vi "Start and End to Array 2.vi"(6 "Sweep Style":enum16{"Linear Step", "Linear Pts", "Log Pts"}(ring), 8 "Round Factor":dbl=1000000000.0, 9 "Step or # Pts":dbl=0.1, 10 "End":dbl=2.0, 11 "Start":dbl=-0.5) -> (3 "Array":dbl[](array[numeric])=[-0.5, -0.4, -0.3, -0.2, -0.1, 0.0, 0.1, 0.2, 0.3, 0.4, 0.5, 0.6, 0.7, 0.8, 0.9, 1.0, 1.1, 1.2, 1.3, 1.4, 1.5, 1.6, 1.7, 1.8, 1.9, 2.0])   [LabVIEW 2010]
panel:
  in  "Array Settings":T1
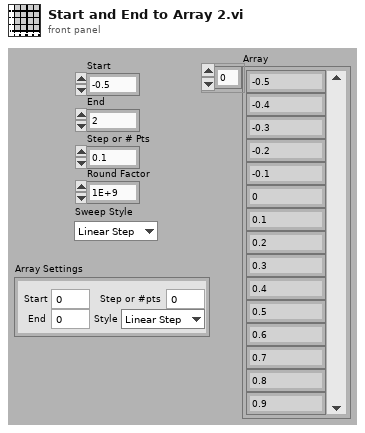
[diagram p1: front panel]
types:
  T1 = cluster{"Start":dbl, "End":dbl, "Step or #pts":dbl, "Style":enum16{"Linear Step", "Linear Pts", "Log Pts"}}
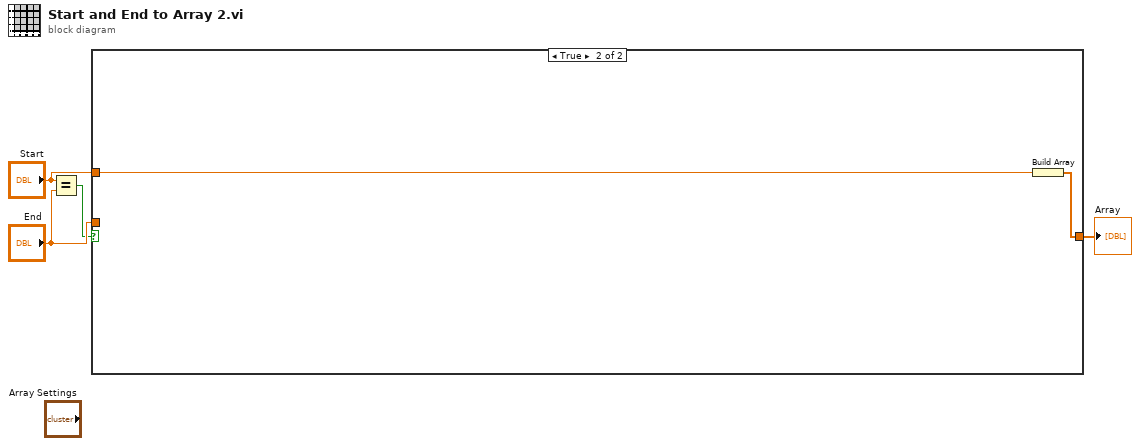
[diagram p0: block diagram]
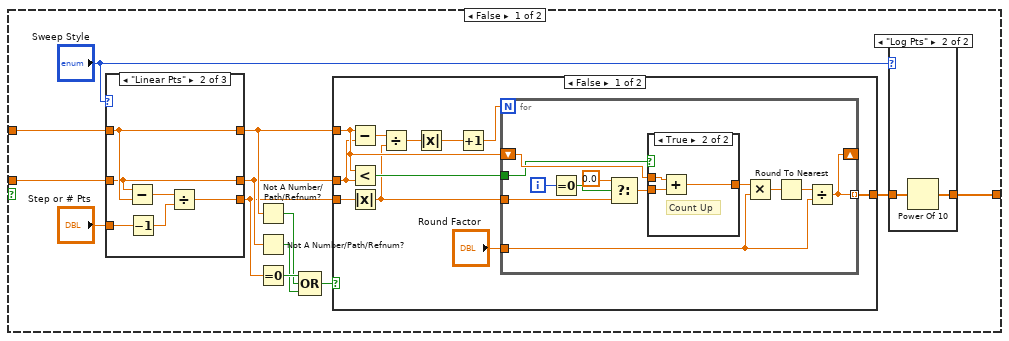
[diagram p2: hidden frame]
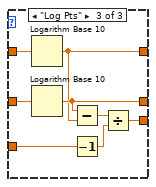
[diagram p5: hidden frame]
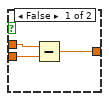
[diagram p6: hidden frame]
diagram:
  n1 = Equal?(x="Start", y="End") -> (x = y?=w2:bool)
  n2 = case shown="True" w2 {
    tunnel: "Start" -> [w13 w68]
    tunnel: "End" -> [w11 _]
    tunnel: [w5 w67] -> w1
    frame False {
      n3 = case shown="\"Linear Pts\"" "Sweep Style" {
        tunnel: w13 -> [w23 w29 w37]
        tunnel: [w23 w29 w33] -> w12
        tunnel: w11 -> [w22 w28 w36]
        tunnel: [w22 w28 w34] -> w10
        tunnel: "Step or # Pts" -> [w21 w25 w31]
        tunnel: [w21 w26 w32] -> w9
        frame "Linear Step", Default {
        }
        frame "Linear Pts" {
          n4 = Subtract(x=w28, y=w29) -> (x-y=w27:dbl)
          n5 = Decrement(x=w25) -> (x-1=w24:dbl)
          n6 = Divide(x=w27, y=w24) -> (x/y=w26:dbl)
        }
        frame "Log Pts" {
          n7 = Logarithm Base 10(1:w37) -> (0:w33:dbl)
          n8 = Logarithm Base 10(1:w36) -> (0:w34:dbl)
          n9 = Subtract(x=w34, y=w33) -> (x-y=w35:dbl)
          n10 = Decrement(x=w31) -> (x-1=w30:dbl)
          n11 = Divide(x=w35, y=w30) -> (x/y=w32:dbl)
        }
      }
      n12 = Not A Number/Path/Refnum?(number/path/refnum=w12) -> (NaN/Path/Refnum?=w16:bool)
      n13 = Not A Number/Path/Refnum?(number/path/refnum=w10) -> (NaN/Path/Refnum?=w15:bool)
      n14 = Equal To 0?(x=w9) -> (x = 0?=w17:bool)
      n15 = Compound Arithmetic op=OR(w17, w16, w15) -> (w14:bool)
      n16 = case shown="False" w14 {
        tunnel: w12 -> [w47 _]
        tunnel: w10 -> [w46 _]
        tunnel: w9 -> [w40 _]
        tunnel: [w38 _] -> w8
        frame False {
          n17 = Subtract(x=w47, y=w46) -> (x-y=w45:dbl)
          n18 = Less?(x=w47, y=w46) -> (x < y?=w48:bool)
          n19 = Absolute Value(x=w40) -> (abs(x)=w39:dbl)
          n20 = Divide(x=w45, y=w39) -> (x/y=w44:dbl)
          n21 = Absolute Value(x=w44) -> (abs(x)=w43:dbl)
          n22 = Increment(x=w43) -> (x+1=w42:dbl)
          n23 = for {
            N: w42 -> [_]
            tunnel: w39 -> [w56]
            tunnel: [w51] -> w38 mode=indexing
            shift-right: [w51] -> _
            shift-left: w47 -> [w60]
            tunnel: "Round Factor" -> [w50]
            tunnel: w48 -> [w49]
            i -> [w59]
            n24 = Equal To 0?(x=w59) -> (x = 0?=w58:bool)
            n25 = Select(t=0.0, s=w58, f=w56) -> (s? t:f=w55:dbl)
            n26 = case shown="True" w49 {
              tunnel: w60 -> [w61 w66]
              tunnel: w55 -> [w63 w65]
              tunnel: [w62 w64] -> w52
              frame False {
                n27 = Subtract(x=w61, y=w63) -> (x-y=w62:dbl)
              }
              frame True {
                # "Count Up"
                n28 = Add(x=w66, y=w65) -> (x+y=w64:dbl)
              }
            }
            n29 = Multiply(x=w52, y=w50) -> (x*y=w54:dbl)
            n30 = Round To Nearest(number=w54) -> (nearest integer value=w53:dbl)
            n31 = Divide(x=w53, y=w50) -> (x/y=w51:dbl)
          }
        }
        frame True {
        }
      }
      n32 = case shown="\"Log Pts\"" "Sweep Style" {
        tunnel: w8 -> [w18 w20]
        tunnel: [w18 w19] -> w5
        frame "Linear Step", Default {
        }
        frame "Log Pts" {
          n33 = Power Of 10(x=w20) -> (10^x=w19:dbl[])
        }
      }
    }
    frame True {
      n34 = Build Array(w68) -> (w67:dbl[])
    }
  }
  "Array" <- w1
